vi "Events to table.vi"(8 "error in (no error)":errorcluster, 11 "object ref in":T1) -> (0 "error out":errorcluster, 2 "table":string[][](array[string]), 3 "object ref out":T1)   [LabVIEW 2013, in "Table Manager.lvlib" / "Table Manager.lvclass"]
uses:
  Table Manager.lvclass
  object ref.ctl
  <vilib>/NI/Tag Bus Data Framework/Configuration Editor/Classes/Engine Parent/Engine Parent Editor Node.lvclass
  <vilib>/NI/Tag Bus Data Framework/Configuration Editor/Classes/Module editor node/module editor node.lvclass
  <vilib>/NI/Tag Bus Module Framework/module configuration/TBM module configuration.lvclass
  <vilib>/NI/Tag Bus Data Framework/Configuration Editor/Classes/Engine Parent/read engine configuration.vi
  <vilib>/NI/Tag Bus Data Framework/Configuration Editor/Classes/Module editor node/Read Module Configuration.vi
  <vilib>/NI/Module Execution Interface/Engine Configuration/engine configuration.lvclass
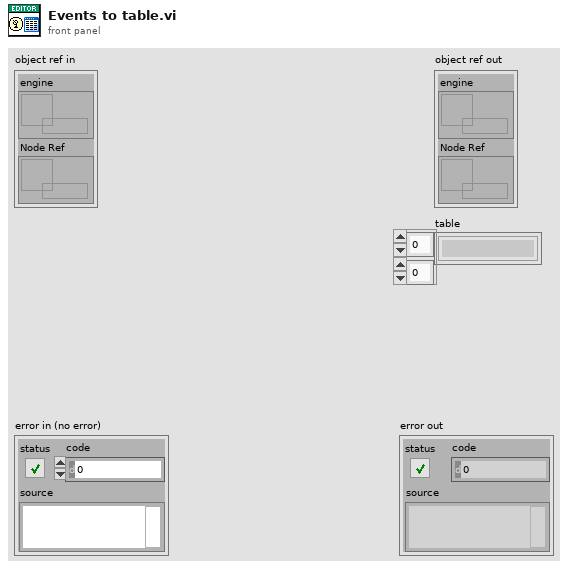
[diagram p1: front panel]
types:
  T1 = typedef "Table Manager.lvlib/Table Manager.lvclass/object ref.ctl" = cluster{"engine":refnum<data-value>, "Node Ref":refnum<data-value>}
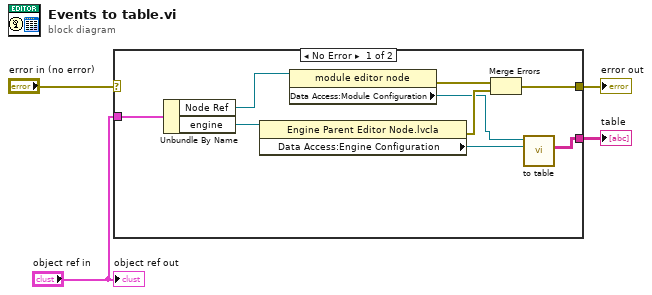
[diagram p0: block diagram]
diagram:
  n1 = case shown="No Error" "error in (no error)" {
    selector: "error in (no error)" -> [_ w14]
    tunnel: [w5 _] -> w4
    tunnel: "object ref in" -> [w11 _]
    tunnel: [w8 w14] -> w1
    frame No Error {
      n2 = Unbundle By Name(w11) -> ("Node Ref"=w12:refnum<data-value>, "engine"=w13:refnum<data-value>)
      n3 = property class="Engine Parent Editor Node.lvcla"(reference=w13) -> (error out=w10:errorcluster, "Data Access:Engine Configuration"=w6:refnum<class "engine configuration.lvclass">)  [unwired: 1 in, 1 out]
      n4 = property class="module editor node"(reference=w12) -> (error out=w9:errorcluster, "Data Access:Module Configuration"=w7:refnum<class "TBM module configuration.lvclass">)  [unwired: 1 in, 1 out]
      n5 = Merge Errors(w9, w10) -> (w8:errorcluster)
      n6 = call-dynamic "to table.vi"("variant"=w6, "configuration in"=w7) -> ("table"=w5:string[][])  [unwired: 7 in, 2 out]
    }
    frame Error {
    }
  }
  "table" <- w4
  "error out" <- w1
  "object ref out" <- "object ref in"
